vi "Create Type Data Clusters (simple).vi"   [LabVIEW 2019]
uses:
  gRPC Template Creation Utility.lvlib
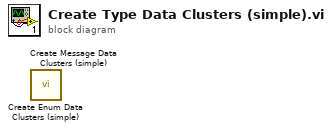
[diagram p0: block diagram]
diagram:
  n1 = call "Create Enum Data Clusters (simple).vi"() -> ()  [unwired: 10 in, 2 out]
  n2 = call "Create Message Data Clusters (simple).vi"() -> ()  [unwired: 10 in, 2 out]
